vi "Initialize DAQ Channel.vi"(8 "error in (no error)":errorcluster, 10 "DAQmx Digital Channel":tag, 11 "DAQ DI in":refnum<class "DAQ DI.lvclass">) -> (0 "error out":errorcluster, 3 "DAQ DI out":refnum<class "DAQ DI.lvclass">)   [LabVIEW 2020, in "DAQ DI.lvlib" / "DAQ DI.lvclass"]
uses:
  DAQ DI.lvclass
  DAQ DI.lvclass/DAQ DI.ctl
  <vilib>/DAQmx/create/channels.llb/DAQmx Create Channel (DI-Digital Input).vi
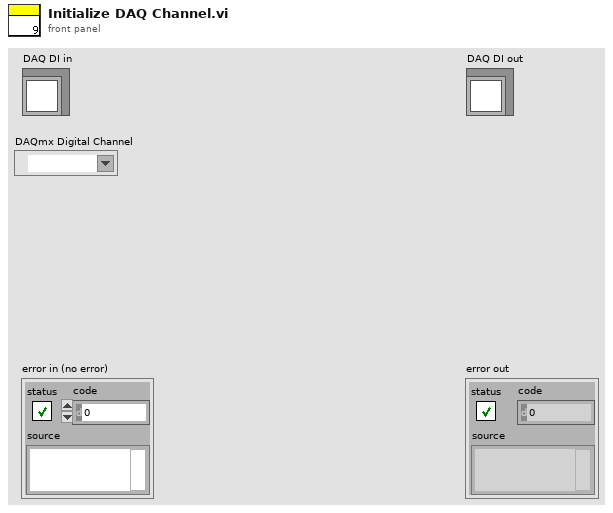
[diagram p1: front panel]
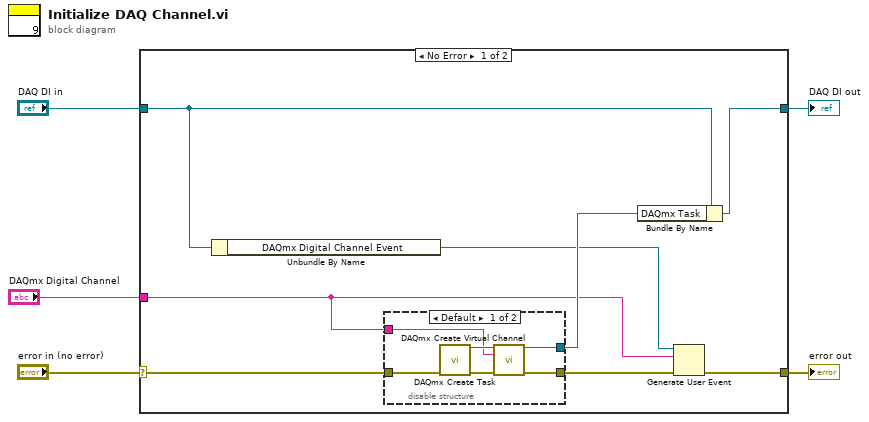
[diagram p0: block diagram]
diagram:
  n1 = case shown="No Error" "error in (no error)" {
    selector: "error in (no error)" -> [w12 w22]
    tunnel: [w7 w22] -> w4
    tunnel: [w13 w21] -> w2
    tunnel: "DAQ DI in" -> [w10 w21]
    tunnel: "DAQmx Digital Channel" -> [w6 _]
    frame No Error {
      n2 = Unbundle By Name(w10) -> ("DAQmx Digital Channel Event"=w9:refnum<user-event>)
      n3 = disable-structure shown="Default" {
        disable-tunnel: w12 -> [w17 w20]
        disable-tunnel: [w16 _] -> w11
        disable-tunnel: [w15 w20] -> w8
        disable-tunnel: w6 -> [w14 _]
        frame condition #0 (active) {
          n4 = call <vilib>:"DAQmx Create Task.vi"("error in"=w17) -> ("task out"=w19:refnum<k21>, "error out"=w18:errorcluster)  [unwired: 13 in]
          n5 = call-poly <vilib>:"DAQmx Create Virtual Channel.vi"("task in"=w19, "lines"=w14, "error in"=w18) -> ("task out"=w16:refnum<k21>, "error out"=w15:errorcluster)  [unwired: 11 in]
        }
        frame condition #1 {
        }
      }
      n6 = Bundle By Name(cluster=w10, "DAQmx Task"=w11) -> (w13:refnum<class "DAQ DI.lvclass">)
      n7 = Generate User Event(user event=w9, event data cluster=w6, error in=w8) -> (error out=w7:errorcluster)  [unwired: 1 in, 1 out]
    }
    frame Error {
    }
  }
  "error out" <- w4
  "DAQ DI out" <- w2
